vi "Table, Scroll to Last Row.vi"(8 "error in":errorcluster, 11 "Tbl Refnum":refnum<vi>) -> (0 "error out":errorcluster, 2 "row_n (I32)":i32=-1, 3 "Tbl Refnum out":refnum<vi>)   [LabVIEW 2010]
doc: "This function scrolls the rows in a table to display the last data row in the last visible table row. The calculation includes an offset for column header visibility."
panel:
  out "row index (U32)":u32
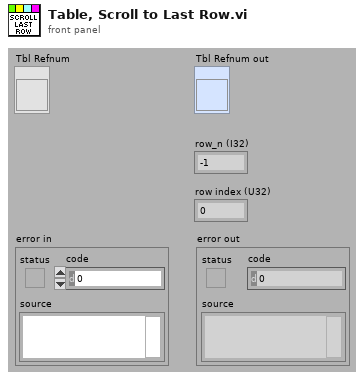
[diagram p1: front panel]
types:
  T1 = typedef "LVRowAndColumnUnsignedTypeDef.ctl" = cluster{"Row":u32, "Column":u32}
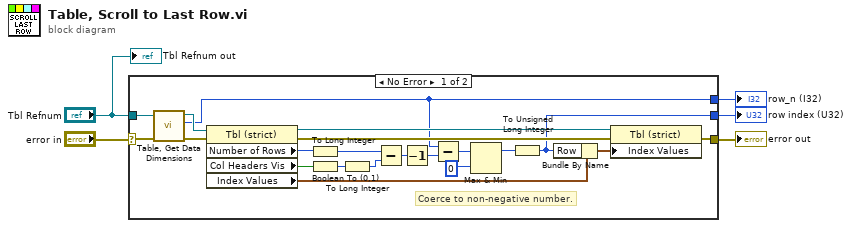
[diagram p0: block diagram]
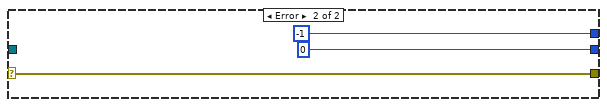
[diagram p2: hidden frame]
diagram:
  n1 = case shown="No Error" "error in" {
    selector: "error in" -> [w22 w29]
    tunnel: "Tbl Refnum" -> [w20 _]
    tunnel: [w16 w29] -> w4
    tunnel: [w9 -1 ("row_n")] -> w2
    tunnel: [w6 u32 0] -> w1
    frame No Error {
      # "Coerce to non-negative number."
      n2 = call "Table, Get Data Dimensions.vi"("error in"=w22, "Tbl Refnum"=w20) -> ("error out"=w21:errorcluster, "row_n"=w9:i32, "Tbl Refnum out"=w19:refnum<vi>)  [unwired: 6 in, 1 out]
      n3 = property class="Tbl (strict)"(reference=w19, error in=w21) -> (reference out=w18:refnum<vi>, error out=w17:errorcluster, "Number of Rows"=w12:u32, "Col Headers Vis"=w23:bool, "Index Values"=w25:T1)
      n4 = To Long Integer(number=w12) -> (32bit integer=w15:i32)
      n5 = Boolean To (0,1)(Boolean=w23) -> (0, 1=w14:i16)
      n6 = To Long Integer(number=w14) -> (32bit integer=w7:i32)
      n7 = Subtract(x=w15, y=w7) -> (x-y=w24:i32)
      n8 = Decrement(x=w24) -> (x-1=w11:i32)
      n9 = Subtract(x=w9, y=w11) -> (x-y=w8:i32)
      n10 = Max & Min(x=w8, y=0 ("lower limit")) -> (max(x,y)=w10:i32)  [unwired: 1 out]
      n11 = To Unsigned Long Integer(number=w10) -> (unsigned 32bit integer=w6:u32)
      n12 = Bundle By Name(cluster=w25, "Row"=w6) -> (w26:T1)
      n13 = property class="Tbl (strict)"(reference=w18, error in=w17, "Index Values"=w26) -> (error out=w16:errorcluster)  [unwired: 1 out]
    }
    frame Error {
    }
  }
  "row_n (I32)" <- w2
  "error out" <- w4
  "row index (U32)" <- w1
  "Tbl Refnum out" <- "Tbl Refnum"
